vi "SaveImageToBmp.vi"(6 "pSrcData":u8[](array[numeric]), 7 "handle":i64, 8 "pDstBuf":u8[](array[numeric]), 9 "fileName":string, 10 "pLbFrame":T1, 11 "error in (no error)":errorcluster) -> (2 "return type":i32, 3 "error out":errorcluster)   [LabVIEW 2016]
uses:
  MVSDKmd.dll
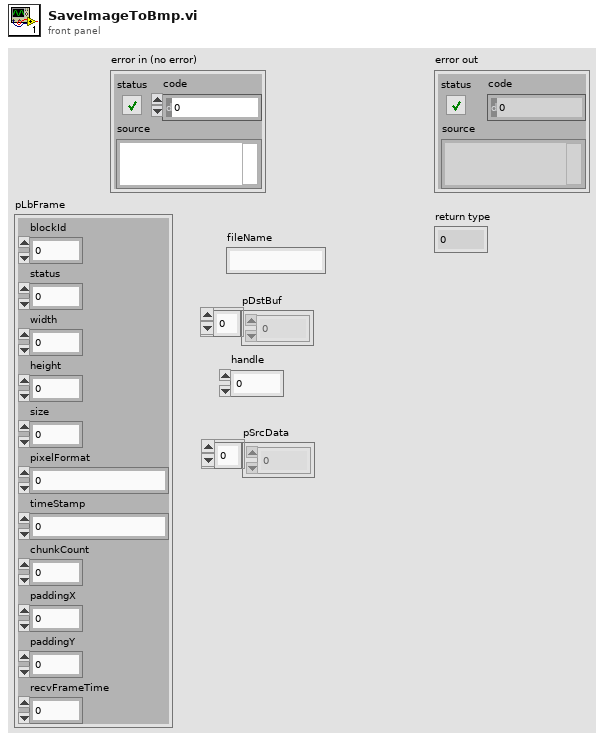
[diagram p1: front panel]
types:
  T1 = cluster{"blockId":u64, "status":u32, "width":u32, "height":u32, "size":u32, "pixelFormat":i32, "timeStamp":u64, "chunkCount":u32, "paddingX":u32, "paddingY":u32, "recvFrameTime":u32}
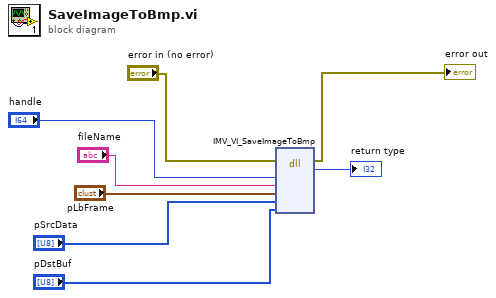
[diagram p0: block diagram]
diagram:
  n1 = dll-call lib="MVSDKmd.dll" fn="IMV_VI_SaveImageToBmp"(error in="error in (no error)", "handle"="handle", "filePath"="fileName", "LbFrame"="pLbFrame", "pSrcData"="pSrcData", "pDstBuf"="pDstBuf") -> (error out=→"error out":errorcluster, "return type"=→"return type":i32)  [unwired: 7 in, 1 out]
